vi "Type to I32.vi"(11 "Voicemeeter Type":T1=enum."Voicemeeter") -> (3 "Type I32":i32)   [LabVIEW 2022 SP3, in "VoiceMeeterRemote.lvlib"]
uses:
  VoiceMeeterRemote.lvlib
  Voicemeeter Type.ctl
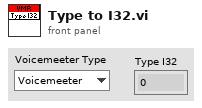
[diagram p1: front panel]
types:
  T1 = typedef "VoiceMeeterRemote.lvlib/Voicemeeter Type.ctl" = enum16{"Unknown", "Voicemeeter", "Banana", "Potato", "Potato x64"}
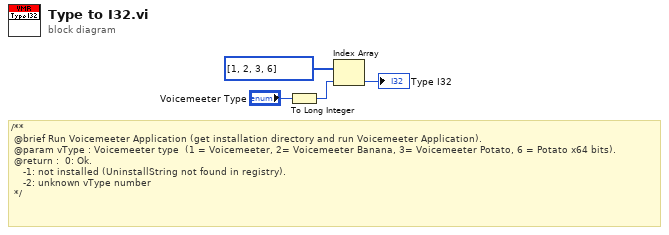
[diagram p0: block diagram]
diagram:
  # "/** \n\t@brief Run Voicemeeter Application (get installation directory and run Voicemeeter Application).\n\t@param vType : Voicemeeter type  (1 = Voicemeeter, 2= Voicemeeter Banana, 3= Voicemeeter Potato, 6 = Potato x64 bits).\n\t@return :\t 0: Ok.\n\t\t\t\t-1: not installed (UninstallString not found in registry).\n\t\t\t\t-2: unknown vType number\n\t*/"
  n1 = To Long Integer(number="Voicemeeter Type") -> (32bit integer=w2:i32)
  n2 = Index Array(array=i32[] [1, 2, 3, 6], index=w2) -> (element=→"Type I32":i32)
